vi "IMG_FORMAT - Type.vi"(8 "error in (no error)":errorcluster, 11 "IMG_FORMAT":T1) -> (0 "error out":errorcluster, 3 "IMG_FORMAT_VALUE":i32)   [LabVIEW 2018]
uses:
  IMG_DATA_FORMAT.ctl
  C:/XIMEA/API/x64/xiApi.NETX64.dll
panel:
  # "Description: Output data format. Notice: image resolution can change after image format has been changed.\nType: Integer.\nDefault: MONO8\nPossible values:\nvalue\tone pixel data in memory [one_byte]\nXI_MONO8\t [Intensity]\nXI_MONO16\t [Intensity LSB] [Intensity MSB]\nXI_RGB24\t [Blue][Green][Red] (Note1)\nXI_RGB32\t [Blue][Green][Red][0]* (Note1)\nXI_RGB_PLANAR\t [Red][Red]...[Green][Green]...[Blue][Blue]... (Note1)\nXI_RAW8\t [pixel byte] raw data from sensor\t\nXI_RAW16\t [pixel byte low] [pixel byte high] 16 bits raw data from sensor\nNote1: Higher CPU processing is required when this mode is selected because color filter array processing is implemented on PC.\nBits alignment: Values are aligned to LSB.\nsensor bits per pixel\tvalues in modes XI_RAW16\n10\t 0-1023\n12\t 0-4095\n14\t 0-16384\nExample: Camera produces 10 bits data and data format XI_RAW16 bit is selected - each 16bit word (pixel) can contain values in range 0-1023"
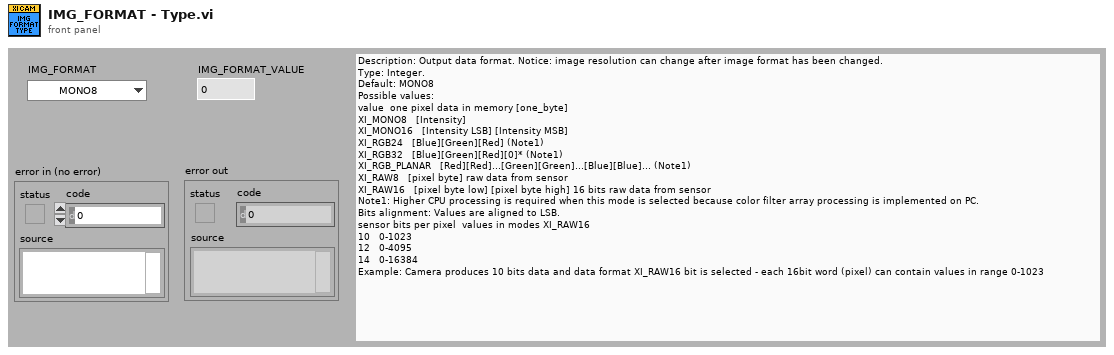
[diagram p1: front panel]
types:
  T1 = typedef "IMG_DATA_FORMAT.ctl" = enum16{"MONO8", "MONO16", "RGB24", "RGB32", "RGBPLANAR", "RAW8", "RAW16"}
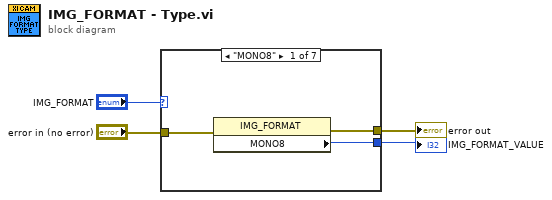
[diagram p0: block diagram]
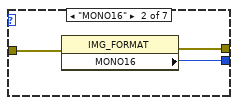
[diagram p2: hidden frame]
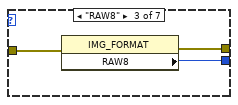
[diagram p3: hidden frame]
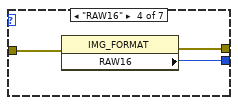
[diagram p4: hidden frame]
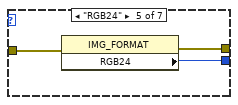
[diagram p5: hidden frame]
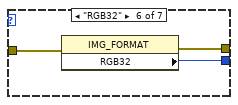
[diagram p6: hidden frame]
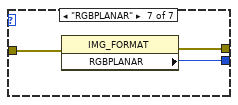
[diagram p7: hidden frame]
diagram:
  n1 = case shown="\"MONO8\"" "IMG_FORMAT" {
    tunnel: "error in (no error)" -> [w7 w10 w13 w16 w19 w22 w25]
    tunnel: [w6 w9 w12 w15 w18 w21 w24] -> w1
    tunnel: [w5 w8 w11 w14 w17 w20 w23] -> w2
    frame "MONO8" {
      n2 = property class="IMG_FORMAT"(error in=w7) -> (error out=w6:errorcluster, "MONO8"=w5:i32)  [unwired: 1 in, 1 out]
    }
    frame "MONO16" {
      n3 = property class="IMG_FORMAT"(error in=w10) -> (error out=w9:errorcluster, "MONO16"=w8:i32)  [unwired: 1 in, 1 out]
    }
    frame "RAW8" {
      n4 = property class="IMG_FORMAT"(error in=w13) -> (error out=w12:errorcluster, "RAW8"=w11:i32)  [unwired: 1 in, 1 out]
    }
    frame "RAW16" {
      n5 = property class="IMG_FORMAT"(error in=w16) -> (error out=w15:errorcluster, "RAW16"=w14:i32)  [unwired: 1 in, 1 out]
    }
    frame "RGB24" {
      n6 = property class="IMG_FORMAT"(error in=w19) -> (error out=w18:errorcluster, "RGB24"=w17:i32)  [unwired: 1 in, 1 out]
    }
    frame "RGB32" {
      n7 = property class="IMG_FORMAT"(error in=w22) -> (error out=w21:errorcluster, "RGB32"=w20:i32)  [unwired: 1 in, 1 out]
    }
    frame "RGBPLANAR" {
      n8 = property class="IMG_FORMAT"(error in=w25) -> (error out=w24:errorcluster, "RGBPLANAR"=w23:i32)  [unwired: 1 in, 1 out]
    }
  }
  "error out" <- w1
  "IMG_FORMAT_VALUE" <- w2
